vi "Lab Panel V5.10.vi"() -> ()   [LabVIEW 2013] (continued)
                n1780 = property on="O/I  LAB05-2" class="Bool (strict)"("DisabledEnum"=w3328) -> ()  [unwired: 2 in, 2 out]
                n1781 = property on="O/I  LAB05-1" class="Bool (strict)"("DisabledEnum"=w3329) -> ()  [unwired: 2 in, 2 out]
                n1782 = property on="O/I  LAB04-1" class="Bool (strict)"("DisabledEnum"=w3331) -> ()  [unwired: 2 in, 2 out]
                n1783 = property on="O/I  LAB04-2" class="Bool (strict)"("DisabledEnum"=w3330) -> ()  [unwired: 2 in, 2 out]
                n1784 = property on="O/I  LAB03-2" class="Bool (strict)"("DisabledEnum"=w3332) -> ()  [unwired: 2 in, 2 out]
                n1785 = Not(x=w3337) -> (.not. x?=w3338:bool)
                n1786 = Not(x=w3336) -> (.not. x?=w3339:bool)
                n1787 = Not(x=w3335) -> (.not. x?=w3340:bool)
                n1788 = property on="RESULT LAB05-2" class="Bool (strict)"("Visible"=w3338) -> ()  [unwired: 2 in, 2 out]
                n1789 = property on="RESULT LAB05-1" class="Bool (strict)"("Visible"=w3339) -> ()  [unwired: 2 in, 2 out]
                n1790 = Not(x=w3334) -> (.not. x?=w3341:bool)
                n1791 = property on="RESULT LAB04-2" class="Bool (strict)"("Visible"=w3340) -> ()  [unwired: 2 in, 2 out]
                n1792 = Not(x=w3333) -> (.not. x?=w3342:bool)
                n1793 = property on="RESULT LAB04-1" class="Bool (strict)"("Visible"=w3341) -> ()  [unwired: 2 in, 2 out]
                n1794 = property on="RESULT LAB03-2" class="Bool (strict)"("Visible"=w3342) -> ()  [unwired: 2 in, 2 out]
              }
              frame #2 {
                # "disable calibrate if any test running"
                n1795 = Or(x=w3365, y=w3364) -> (x .or. y?=w3358:bool)
                n1796 = Or(x=w3367, y=w3366) -> (x .or. y?=w3360:bool)
                n1797 = Or(x=w3371, y=w3370) -> (x .or. y?=w3362:bool)
                n1798 = Or(x=w3369, y=w3368) -> (x .or. y?=w3361:bool)
                n1799 = Or(x=w3373, y=w3372) -> (x .or. y?=w3363:bool)
                n1800 = Or(x=w3361, y=w3360) -> (x .or. y?=w3359:bool)
                n1801 = Or(x=w3363, y=w3362) -> (x .or. y?=w3357:bool)
                n1802 = Or(x=w3359, y=w3358) -> (x .or. y?=w3356:bool)
                n1803 = Or(x=w3357, y=w3356) -> (x .or. y?=w3355:bool)
                n1804 = case shown="False" w3355 {
                  tunnel: [0 2] -> w3354
                  frame False {
                  }
                  frame True {
                  }
                }
                n1805 = property on="JIG TEST" class="Clust (strict)"("DisabledEnum"=w3354) -> ()  [unwired: 2 in, 2 out]
                n1806 = property on="Network Directory" class="Path"("DisabledEnum"=w3354) -> ()  [unwired: 2 in, 2 out]
                n1807 = property on="MAIL SETTINGS" class="Clust (strict)"("DisabledEnum"=w3354) -> ()  [unwired: 2 in, 2 out]
                n1808 = property on="SET (cal)" class="Bool (strict)"("DisabledEnum"=w3354) -> ()  [unwired: 2 in, 2 out]
                n1809 = property on="ADMIN" class="Bool (strict)"("DisabledEnum"=0) -> ()  [unwired: 2 in, 2 out]
              }
            }
          }
          frame #8 {
            # "drive jigs"
            n1810 = stacked-sequence {
              frame #0 {
                # "jig on"
                n1811 = local read "jig cycle"() -> (w3381:dbl)
                n1812 = property on="JIG TEST" class="Clust (strict)"() -> ("DisabledEnum"=w3378:T16)  [unwired: 2 in, 2 out]
                n1813 = Equal?(x=w3378, y=2) -> (x = y?=w3377:bool)
                n1814 = Equal?(x=w3381, y=0) -> (x = y?=w3379:bool)
                n1815 = And(x=w3379, y=w3377) -> (x .and. y?=w3376:bool)
                n1816 = case shown="True" w3376 {
                  frame False {
                  }
                  frame True {
                    n1817 = local read "run lab01-1"() -> (w3392:bool)
                    n1818 = local read "run lab01-2"() -> (w3391:bool)
                    n1819 = local read "run lab02-1"() -> (w3390:bool)
                    n1820 = local read "run lab02-2"() -> (w3389:bool)
                    n1821 = local read "run lab03-1"() -> (w3388:bool)
                    n1822 = local read "run lab03-2"() -> (w3387:bool)
                    n1823 = local read "run lab04-1"() -> (w3386:bool)
                    n1824 = local read "run lab04-2"() -> (w3385:bool)
                    n1825 = local read "run lab05-1"() -> (w3384:bool)
                    n1826 = local read "run lab05-2"() -> (w3383:bool)
                    n1827 = local write "JIG LAB03-2"(w3387) -> ()
                    n1828 = local write "JIG LAB01-1"(w3392) -> ()
                    n1829 = local write "JIG LAB01-2"(w3391) -> ()
                    n1830 = local write "JIG LAB02-1"(w3390) -> ()
                    n1831 = local write "JIG LAB02-2"(w3389) -> ()
                    n1832 = local write "JIG LAB03-1"(w3388) -> ()
                    n1833 = local write "JIG LAB04-1"(w3386) -> ()
                    n1834 = local write "JIG LAB04-2"(w3385) -> ()
                    n1835 = local write "JIG LAB05-1"(w3384) -> ()
                    n1836 = local write "JIG LAB05-2"(w3383) -> ()
                  }
                }
              }
              frame #1 {
                # "jig off"
                n1837 = local read "jig cycle"() -> (w3399:dbl)
                n1838 = local read "on loops"() -> (w3398:dbl)
                n1839 = property on="JIG TEST" class="Clust (strict)"() -> ("DisabledEnum"=w3397:T16)  [unwired: 2 in, 2 out]
                n1840 = Equal?(x=w3397, y=2) -> (x = y?=w3395:bool)
                n1841 = Equal?(x=w3399, y=w3398) -> (x = y?=w3394:bool)
                n1842 = And(x=w3394, y=w3395) -> (x .and. y?=w3393:bool)
                n1843 = case shown="True" w3393 {
                  frame False {
                  }
                  frame True {
                    w3450 = FALSE
                    w3451 = TRUE
                    w3449 = 2
                    n1844 = local read "SELECT LAB05-2"() -> (w3440:T3)
                    n1845 = local read "SELECT LAB04-2"() -> (w3442:T3)
                    n1846 = local read "SELECT LAB04-1"() -> (w3443:T3)
                    n1847 = local read "SELECT LAB05-1"() -> (w3441:T3)
                    n1848 = local read "SELECT LAB03-2"() -> (w3444:T3)
                    n1849 = local read "SELECT LAB02-1"() -> (w3447:T3)
                    n1850 = local read "SELECT LAB03-1"() -> (w3445:T3)
                    n1851 = local read "SELECT LAB02-2"() -> (w3446:T3)
                    n1852 = local read "SELECT LAB01-2"() -> (w3448:T3)
                    n1853 = local read "run lab05-1"() -> (w3410:bool)
                    n1854 = local read "run lab05-2"() -> (w3409:bool)
                    n1855 = local read "SELECT LAB01-1"() -> (w3452:T3)
                    n1856 = local read "run lab04-2"() -> (w3411:bool)
                    n1857 = local read "run lab04-1"() -> (w3412:bool)
                    n1858 = local read "run lab01-1"() -> (w3428:bool)
                    n1859 = local read "run lab01-2"() -> (w3417:bool)
                    n1860 = local read "run lab03-2"() -> (w3413:bool)
                    n1861 = local read "run lab03-1"() -> (w3414:bool)
                    n1862 = local read "run lab02-1"() -> (w3416:bool)
                    n1863 = local read "run lab02-2"() -> (w3415:bool)
                    n1864 = Equal?(x=w3449, y=w3445) -> (x = y?=w3423:bool)
                    n1865 = Equal?(x=w3449, y=w3444) -> (x = y?=w3422:bool)
                    n1866 = Equal?(x=w3449, y=w3443) -> (x = y?=w3421:bool)
                    n1867 = Equal?(x=w3449, y=w3442) -> (x = y?=w3420:bool)
                    n1868 = Equal?(x=w3449, y=w3441) -> (x = y?=w3419:bool)
                    n1869 = Equal?(x=w3449, y=w3440) -> (x = y?=w3418:bool)
                    n1870 = Equal?(x=w3449, y=w3452) -> (x = y?=w3429:bool)
                    n1871 = Equal?(x=w3449, y=w3447) -> (x = y?=w3425:bool)
                    n1872 = Equal?(x=w3449, y=w3446) -> (x = y?=w3424:bool)
                    n1873 = Equal?(x=w3449, y=w3448) -> (x = y?=w3426:bool)
                    n1874 = And(x=w3420, y=w3411) -> (x .and. y?=w3402:bool)
                    n1875 = And(x=w3423, y=w3414) -> (x .and. y?=w3405:bool)
                    n1876 = And(x=w3421, y=w3412) -> (x .and. y?=w3403:bool)
                    n1877 = And(x=w3418, y=w3409) -> (x .and. y?=w3400:bool)
                    n1878 = And(x=w3424, y=w3415) -> (x .and. y?=w3406:bool)
                    n1879 = And(x=w3422, y=w3413) -> (x .and. y?=w3404:bool)
                    n1880 = And(x=w3419, y=w3410) -> (x .and. y?=w3401:bool)
                    n1881 = And(x=w3426, y=w3417) -> (x .and. y?=w3408:bool)
                    n1882 = And(x=w3429, y=w3428) -> (x .and. y?=w3427:bool)
                    n1883 = And(x=w3425, y=w3416) -> (x .and. y?=w3407:bool)
                    n1884 = Select(t=w3451, s=w3427, f=w3450) -> (s? t:f=w3430:bool)
                    n1885 = Select(t=w3451, s=w3408, f=w3450) -> (s? t:f=w3431:bool)
                    n1886 = Select(t=w3451, s=w3407, f=w3450) -> (s? t:f=w3432:bool)
                    n1887 = Select(t=w3451, s=w3406, f=w3450) -> (s? t:f=w3433:bool)
                    n1888 = Select(t=w3451, s=w3405, f=w3450) -> (s? t:f=w3434:bool)
                    n1889 = Select(t=w3451, s=w3404, f=w3450) -> (s? t:f=w3435:bool)
                    n1890 = Select(t=w3451, s=w3403, f=w3450) -> (s? t:f=w3436:bool)
                    n1891 = Select(t=w3451, s=w3402, f=w3450) -> (s? t:f=w3437:bool)
                    n1892 = Select(t=w3451, s=w3401, f=w3450) -> (s? t:f=w3438:bool)
                    n1893 = Select(t=w3451, s=w3400, f=w3450) -> (s? t:f=w3439:bool)
                    n1894 = local write "JIG LAB03-2"(w3435) -> ()
                    n1895 = local write "JIG LAB02-1"(w3432) -> ()
                    n1896 = local write "JIG LAB02-2"(w3433) -> ()
                    n1897 = local write "JIG LAB01-2"(w3431) -> ()
                    n1898 = local write "JIG LAB03-1"(w3434) -> ()
                    n1899 = local write "JIG LAB01-1"(w3430) -> ()
                    n1900 = local write "JIG LAB05-2"(w3439) -> ()
                    n1901 = local write "JIG LAB04-1"(w3436) -> ()
                    n1902 = local write "JIG LAB05-1"(w3438) -> ()
                    n1903 = local write "JIG LAB04-2"(w3437) -> ()
                  }
                }
              }
            }
          }
          frame #9 {
            # "enable  jig test output if no test busy"
            n1904 = property on="JIG TEST" class="Clust (strict)"() -> ("DisabledEnum"=w3455:T16)  [unwired: 2 in, 2 out]
            n1905 = Equal?(x=w3455, y=0) -> (x = y?=w3453:bool)
            n1906 = case shown="True" w3453 {
              frame False {
              }
              frame True {
                n1907 = local read "JIG TEST"() -> (w3466:T10)
                n1908 = Unbundle(w3466) -> ("LAB01-1"=w3465:bool, "LAB01-2"=w3464:bool, "LAB02-1"=w3463:bool, "LAB02-2"=w3462:bool, "LAB03-1"=w3461:bool, "LAB03-2"=w3460:bool, "LAB04-1"=w3459:bool, "LAB04-2"=w3458:bool, "LAB05-1"=w3457:bool, "LAB05-2"=w3456:bool)
                n1909 = local write "JIG LAB05-1"(w3457) -> ()
                n1910 = local write "JIG LAB05-2"(w3456) -> ()
                n1911 = local write "JIG LAB04-1"(w3459) -> ()
                n1912 = local write "JIG LAB04-2"(w3458) -> ()
                n1913 = local write "JIG LAB03-2"(w3460) -> ()
                n1914 = local write "JIG LAB01-1"(w3465) -> ()
                n1915 = local write "JIG LAB02-1"(w3463) -> ()
                n1916 = local write "JIG LAB03-1"(w3461) -> ()
                n1917 = local write "JIG LAB01-2"(w3464) -> ()
                n1918 = local write "JIG LAB02-2"(w3462) -> ()
              }
            }
          }
          frame #10 {
            # "Drive digital output and reset USB and temperature network if required."
            n1919 = global read "Global display 3.vi" "cycle O/F"() -> (w3477:bool)
            n1920 = local read "O/I  LAB05-2"() -> (w3470:bool)
            n1921 = local read "O/I  LAB05-1"() -> (w3472:bool)
            n1922 = local read "JIG LAB05-2"() -> (w3469:bool)
            n1923 = local read "O/I  LAB04-2"() -> (w3474:bool)
            n1924 = local read "JIG LAB05-1"() -> (w3471:bool)
            n1925 = local read "JIG LAB04-2"() -> (w3473:bool)
            n1926 = local read "O/I  LAB03-1"() -> (w3488:bool)
            n1927 = local read "O/I  LAB04-1"() -> (w3484:bool)
            n1928 = local read "O/I  LAB02-1"() -> (w3492:bool)
            n1929 = local read "O/I  LAB02-2"() -> (w3490:bool)
            n1930 = local read "O/I  LAB03-2"() -> (w3486:bool)
            n1931 = local read "JIG LAB04-1"() -> (w3483:bool)
            n1932 = local read "JIG LAB03-2"() -> (w3485:bool)
            n1933 = local read "O/I  LAB01-2"() -> (w3494:bool)
            n1934 = local read "JIG LAB02-1"() -> (w3491:bool)
            n1935 = local read "JIG LAB02-2"() -> (w3489:bool)
            n1936 = local read "JIG LAB03-1"() -> (w3487:bool)
            n1937 = local read "O/I  LAB01-1"() -> (w3496:bool)
            n1938 = local read "JIG LAB01-2"() -> (w3493:bool)
            n1939 = local read "JIG LAB01-1"() -> (w3495:bool)
            n1940 = case shown="False" w3477 {
              tunnel: [w3542 FALSE] -> w3476
              frame False {
                n1941 = local read "Analog error"() -> (w3541:bool)
                n1942 = local read "Reset Measuring"() -> (w3540:bool)
                n1943 = Or(x=w3540, y=w3541) -> (x .or. y?=w3542:bool)
              }
              frame True {
              }
            }
            n1944 = Build Array(w3489, w3488, w3487, w3486, w3485, w3484, w3483) -> (w3481:bool[])
            n1945 = Build Array(w3496, w3495, w3494, w3493, w3492, w3491, w3490) -> (w3482:bool[])
            n1946 = Build Array(w3474, w3473, w3472, w3471, w3470, w3469, w3476) -> (w3480:bool[])
            n1947 = Build Array(w3474, w3473, w3472, w3471, w3470, w3469, FALSE) -> (w3467:bool[])
            n1948 = Not(x=w3477) -> (.not. x?=w3478:bool)
            n1949 = local read "simulate"() -> (w3479:bool)
            n1950 = And(x=w3478, y=w3476) -> (x .and. y?=w3475:bool)
            n1951 = stacked-sequence {
              tunnel: w3482 -> [w3500 w3506]
              tunnel: w3481 -> [w3499 w3505]
              tunnel: w3480 -> [w3498 _]
              tunnel: w3479 -> [w3497 w3507]
              tunnel: w3475 -> [_ w3508]
              tunnel: w3467 -> [_ w3504]
              frame #0 {
                n1952 = case shown="False" w3497 {
                  tunnel: w3500 -> [w3503 _]
                  tunnel: w3499 -> [w3502 _]
                  tunnel: w3498 -> [w3501 _]
                  frame False {
                    n1953 = call "sub vi - Drive Relays All v6.vi"("Array #2"=w3501, "Array #1"=w3502, "Array #0"=w3503) -> ()  [unwired: 8 in, 1 out]
                  }
                  frame True {
                  }
                }
              }
              frame #1 {
                n1954 = case shown="True" w3508 {
                  tunnel: w3507 -> [_ w3513]
                  tunnel: w3506 -> [_ w3511]
                  tunnel: w3505 -> [_ w3510]
                  tunnel: w3504 -> [_ w3509]
                  frame False {
                  }
                  frame True {
                    n1955 = stacked-sequence {
                      tunnel: w3513 -> [w3520 _]
                      tunnel: bool[] [] -> [_ w3525]
                      tunnel: w3511 -> [_ w3524]
                      tunnel: w3510 -> [_ w3522]
                      tunnel: w3509 -> [_ w3521]
                      frame #0 {
                        w3516 = FALSE
                        # "reset all usb modules"
                        n1956 = local read "Resets Done"() -> (w3515:dbl)
                        n1957 = call "Reset Meas v 3.vi"("simulate"=w3520) -> ("Error USB #2"=w3517:bool, "Error USB #1"=w3518:bool, "Error USB #0"=w3519:bool)  [unwired: 8 in]
                        n1958 = Increment(x=w3515) -> (x+1=→"Resets Done":dbl)
                        n1959 = local write "Error USB #2"(w3517) -> ()
                        n1960 = local write "Error USB #0"(w3519) -> ()
                        n1961 = local write "Error USB #1"(w3518) -> ()
                        n1962 = local write "Reset Measuring"(w3516) -> ()
                        n1963 = local write "Analog error"(w3516) -> ()
                      }
                      frame #1 {
                        # "switch test stations back on after reset"
                        n1964 = stacked-sequence {
                          tunnel: w3525 -> [w3529 w3532 _]
                          tunnel: w3524 -> [w3528 w3534 w3539]
                          tunnel: 3000 -> [w3527 w3530 w3535]
                          tunnel: w3522 -> [_ w3533 w3538]
                          tunnel: w3521 -> [_ _ w3537]
                          frame #0 {
                            # "drive 1st 7 inputs"
                            n1965 = call "sub vi - Drive Relays All v6.vi"("Array #2"=w3529, "Array #1"=w3529, "Array #0"=w3528) -> ()  [unwired: 8 in, 1 out]
                            n1966 = call "Message Display V1.vi"("Message"="Delay on LAB 01-1 to 02-1", "Delay mS"=w3527) -> ()  [unwired: 10 in]
                          }
                          frame #1 {
                            # "drive 1st & 2nd outputs"
                            n1967 = call "sub vi - Drive Relays All v6.vi"("Array #2"=w3532, "Array #1"=w3533, "Array #0"=w3534) -> ()  [unwired: 8 in, 1 out]
                            n1968 = call "Message Display V1.vi"("Message"="Delay on LAB 02-2 to 04-1", "Delay mS"=w3530) -> ()  [unwired: 10 in]
                          }
                          frame #2 {
                            n1969 = call "sub vi - Drive Relays All v6.vi"("Array #2"=w3537, "Array #1"=w3538, "Array #0"=w3539) -> ()  [unwired: 8 in, 1 out]
                            n1970 = call "Message Display V1.vi"("Message"="Delay on LAB 04-2 to 05-2", "Delay mS"=w3535) -> ()  [unwired: 10 in]
                          }
                        }
                      }
                    }
                  }
                }
              }
            }
          }
          frame #11 {
            # "get all analog values from USB devices"
            n1971 = local read "on loops"() -> (w3550:dbl)
            n1972 = local read "jig cycle"() -> (w3547:dbl)
            n1973 = Add(x=w3550, y=1) -> (x+y=w3548:dbl)
            n1974 = Equal?(x=w3547, y=1) -> (x = y?=w3544:bool)
            n1975 = Equal?(x=w3547, y=w3548) -> (x = y?=w3546:bool)
            n1976 = Or(x=w3544, y=w3546) -> (x .or. y?=w3545:bool)
            n1977 = global write "Global display 3.vi" "cycle O/F"(w3544) -> ()
            n1978 = case shown="True" w3545 {
              tunnel: w3544 -> [_ w3554]
              frame False {
              }
              frame True {
                n1979 = local read "simulate"() -> (w3557:bool)
                n1980 = case shown="False" w3557 {
                  tunnel: [w3573 0.3 ("Analog loop time")] -> w3564
                  tunnel: [w3572 dynamicdata[] [] ("array GRAPH")] -> w3563
                  tunnel: [w3571 w3578] -> w3562
                  tunnel: [w3570 w3578] -> w3561
                  tunnel: [w3569 w3578] -> w3560
                  tunnel: [w3568 w3578] -> w3559
                  tunnel: [w3567 w3578] -> w3558
                  tunnel: w3554 -> [_ w3582]
                  tunnel: [w3566 "Ambient Volts"] -> w3553
                  tunnel: [w3565 bool[] []] -> w3552
                  frame False {
                    n1981 = call "sub vi - Read Analog All v9.2.vi"() -> ("Analog loop time"=w3573:dbl, "array GRAPH"=w3572:dynamicdata[], "LAB01"=w3571:T26, "LAB02"=w3570:T27, "LAB03"=w3569:T28, "LAB04"=w3568:T29, "deg C"=w3566:dbl, "USB Error"=w3565:bool[], "LAB05"=w3567:T30)  [unwired: 7 in]
                  }
                  frame True {
                    n1982 = local read "ON amps"() -> (w3576:dbl)
                    n1983 = local read "OFF amps"() -> (w3577:dbl)
                    n1984 = local read "VOLTS"() -> (w3580:dbl)
                    n1985 = local read "PF"() -> (w3579:dbl)
                    n1986 = Select(t=w3576, s=w3582, f=w3577) -> (s? t:f=w3581:dbl)
                    n1987 = Bundle("OFF amps"=w3581, "VOLTS"=w3580, "PF"=w3579, "OFF amps"=w3581, "VOLTS"=w3580, "PF"=w3579) -> (w3578:T31)  [unwired: 1 in]
                  }
                }
                n1988 = local read "simulate"() -> (w3556:bool)
                n1989 = stacked-sequence {
                  tunnel: w3564 -> [w3597 _ _ _ _ _ _]
                  tunnel: w3563 -> [w3594 _ _ _ _ _ _]
                  tunnel: w3562 -> [_ w3644 _ _ _ _ _]
                  tunnel: w3561 -> [_ _ w3651 _ _ _ _]
                  tunnel: w3560 -> [_ _ _ w3680 _ _ _]
                  tunnel: w3559 -> [_ _ _ _ w3707 _ _]
                  tunnel: w3558 -> [_ _ _ _ _ w3736 _]
                  tunnel: w3556 -> [_ w3622 w3650 w3678 w3706 w3734 w3765]
                  tunnel: T14 {"1  (A) cal"=1.0, "1 (V) cal"=1.0, "1 (PF) cal"=1.0, "1 (TL) cal"=1.0, "1 (TN) cal"=1.0, "2 (A) cal"=1.0, "2 (V) cal"=1.0, "2 (PF) cal"=1.0, "2 (TL) cal"=1.0, "2 (TN) cal"=1.0} ("CAL LAB01") -> [_ w3621 w3649 w3677 w3705 w3733 _]
                  tunnel: w3553 -> [_ _ _ _ _ _ w3763]
                  tunnel: w3552 -> [w3593 _ _ _ _ _ _]
                  frame #0 {
                    n1990 = Index Array(array=w3593, index=2) -> (element=w3586:bool)
                    n1991 = Index Array(array=w3593, index=1) -> (element=w3588:bool)
                    n1992 = Index Array(array=w3593, index=0) -> (element=w3589:bool)
                    n1993 = local write "AI"(TRUE) -> ()
                    n1994 = Or(x=w3589, y=w3588) -> (x .or. y?=w3587:bool)
                    n1995 = local write "Error USB #2"(w3586) -> ()
                    n1996 = local write "Error USB #0"(w3589) -> ()
                    n1997 = local write "Error USB #1"(w3588) -> ()
                    n1998 = Or(x=w3587, y=w3586) -> (x .or. y?=→"Analog error":bool)
                    n1999 = global write "Global 1.vi" "RATE(Hz)"("RATE (Hz)") -> ()
                    n2000 = global write "Global 1.vi" "SAMPLES"("SAMPLES") -> ()
                    n2001 = Index Array(array=w3594, index=6) -> (element=→"LAB04-1 (GRAPH)":dynamicdata)
                    n2002 = Index Array(array=w3594, index=7) -> (element=→"LAB04-2 (GRAPH)":dynamicdata)
                    n2003 = Index Array(array=w3594, index=9) -> (element=→"LAB05-2 (GRAPH)":dynamicdata)
                    n2004 = Index Array(array=w3594, index=8) -> (element=→"LAB05-1 (GRAPH)":dynamicdata)
                    n2005 = Index Array(array=w3594, index=5) -> (element=→"LAB03-2 (GRAPH)":dynamicdata)
                    n2006 = Index Array(array=w3594, index=0) -> (element=→"LAB01-1 (GRAPH)":dynamicdata)
                    n2007 = Index Array(array=w3594, index=1) -> (element=→"LAB01-2 (GRAPH)":dynamicdata)
                    n2008 = Index Array(array=w3594, index=2) -> (element=→"LAB02-1 (GRAPH)":dynamicdata)
                    n2009 = Index Array(array=w3594, index=3) -> (element=→"LAB02-2 (GRAPH)":dynamicdata)
                    n2010 = Index Array(array=w3594, index=4) -> (element=→"LAB03-1 (GRAPH)":dynamicdata)
                    "AI loop time" <- w3597
                  }
                  frame #1 {
                    n2011 = case shown="False" w3622 {
                      tunnel: [w3645 w3646] -> w3643
                      tunnel: w3621 -> [_ w3646]
                      frame False {
                        n2012 = local read "CAL LAB01"() -> (w3645:T14)
                      }
                      frame True {
                      }
                    }
                    n2013 = Unbundle By Name(w3644) -> ("OFF amps"=w3642:dbl, "VOLTS"=w3641:dbl, "PF"=w3640:dbl, "OFF amps"=w3639:dbl, "VOLTS"=w3638:dbl, "PF"=w3637:dbl)
                    n2014 = Unbundle By Name(w3643) -> ("1  (A) cal"=w3636:dbl, "1 (V) cal"=w3635:dbl, "1 (PF) cal"=w3634:dbl, "2 (A) cal"=w3633:dbl, "2 (V) cal"=w3632:dbl, "2 (PF) cal"=w3631:dbl)  [unwired: 4 out]
                    n2015 = Multiply(x=w3642, y=w3636) -> (x*y=w3629:dbl)
                    n2016 = Multiply(x=w3641, y=w3635) -> (x*y=w3628:dbl)
                    n2017 = Multiply(x=w3640, y=w3634) -> (x*y=w3627:dbl)
                    n2018 = Multiply(x=w3639, y=w3633) -> (x*y=w3625:dbl)
                    n2019 = Multiply(x=w3638, y=w3632) -> (x*y=w3624:dbl)
                    n2020 = Multiply(x=w3637, y=w3631) -> (x*y=w3623:dbl)
                    n2021 = local read "SIG LAB01-1"() -> (w3630:T2)
                    n2022 = local read "SIG LAB01-2"() -> (w3626:T2)
                    n2023 = Bundle By Name(cluster=w3630, "AMPS"=w3629, "VOLTS"=w3628, "PF"=w3627) -> (w3620:T2)
                    n2024 = Bundle By Name(cluster=w3626, "AMPS"=w3625, "VOLTS"=w3624, "PF"=w3623) -> (w3619:T2)
                    n2025 = global write "Global display 1.vi" "SIG LAB01-2"(w3619) -> ()
                    n2026 = global write "Global display 1.vi" "SIG LAB01-1"(w3620) -> ()
                    n2027 = local write "SIG LAB01-2"(w3619) -> ()
                    n2028 = local write "SIG LAB01-1"(w3620) -> ()
                  }
                  frame #2 {
                    n2029 = Unbundle By Name(w3651) -> ("OFF amps"=w3671:dbl, "VOLTS"=w3670:dbl, "PF"=w3669:dbl, "OFF amps"=w3668:dbl, "VOLTS"=w3667:dbl, "PF"=w3666:dbl)
                    n2030 = case shown="True" w3650 {
                      tunnel: [w3673 w3674] -> w3672
                      tunnel: w3649 -> [_ w3674]
                      frame False {
                        n2031 = local read "CAL LAB02"() -> (w3673:T15)
                      }
                      frame True {
                      }
                    }
                    n2032 = Unbundle By Name(w3672) -> ("1  (A) cal"=w3665:dbl, "1 (V) cal"=w3664:dbl, "1 (PF) cal"=w3663:dbl, "2 (A) cal"=w3662:dbl, "2 (V) cal"=w3661:dbl, "2 (PF) cal"=w3660:dbl)  [unwired: 4 out]
                    n2033 = Multiply(x=w3671, y=w3665) -> (x*y=w3658:dbl)
                    n2034 = Multiply(x=w3670, y=w3664) -> (x*y=w3657:dbl)
                    n2035 = Multiply(x=w3669, y=w3663) -> (x*y=w3656:dbl)
                    n2036 = Multiply(x=w3668, y=w3662) -> (x*y=w3654:dbl)
                    n2037 = Multiply(x=w3667, y=w3661) -> (x*y=w3653:dbl)
                    n2038 = Multiply(x=w3666, y=w3660) -> (x*y=w3652:dbl)
                    n2039 = local read "SIG LAB02-1"() -> (w3659:T2)
                    n2040 = local read "SIG LAB02-2"() -> (w3655:T2)
                    n2041 = Bundle By Name(cluster=w3659, "AMPS"=w3658, "VOLTS"=w3657, "PF"=w3656) -> (w3648:T2)
                    n2042 = Bundle By Name(cluster=w3655, "AMPS"=w3654, "VOLTS"=w3653, "PF"=w3652) -> (w3647:T2)
                    n2043 = global write "Global display 1.vi" "SIG LAB02-1"(w3648) -> ()
                    n2044 = local write "SIG LAB02-2"(w3647) -> ()
                    n2045 = global write "Global display 1.vi" "SIG LAB02-2"(w3647) -> ()
                    n2046 = local write "SIG LAB02-1"(w3648) -> ()
                  }
                  frame #3 {
                    n2047 = Unbundle By Name(w3680) -> ("OFF amps"=w3699:dbl, "VOLTS"=w3698:dbl, "PF"=w3697:dbl, "OFF amps"=w3696:dbl, "VOLTS"=w3695:dbl, "PF"=w3694:dbl)
                    n2048 = case shown="True" w3678 {
                      tunnel: [w3701 w3702] -> w3700
                      tunnel: w3677 -> [_ w3702]
                      frame False {
                        n2049 = local read "CAL LAB03"() -> (w3701:T14)
                      }
                      frame True {
                      }
                    }
                    n2050 = Unbundle By Name(w3700) -> ("1  (A) cal"=w3693:dbl, "1 (V) cal"=w3692:dbl, "1 (PF) cal"=w3691:dbl, "2 (A) cal"=w3690:dbl, "2 (V) cal"=w3689:dbl, "2 (PF) cal"=w3688:dbl)  [unwired: 4 out]
                    n2051 = Multiply(x=w3699, y=w3693) -> (x*y=w3686:dbl)
                    n2052 = Multiply(x=w3698, y=w3692) -> (x*y=w3679:dbl)
                    n2053 = Multiply(x=w3697, y=w3691) -> (x*y=w3685:dbl)
                    n2054 = Multiply(x=w3696, y=w3690) -> (x*y=w3683:dbl)
                    n2055 = Multiply(x=w3695, y=w3689) -> (x*y=w3682:dbl)
                    n2056 = Multiply(x=w3694, y=w3688) -> (x*y=w3681:dbl)
                    n2057 = local read "SIG LAB03-1"() -> (w3687:T2)
                    n2058 = local read "SIG LAB03-2"() -> (w3684:T2)
                    n2059 = Bundle By Name(cluster=w3687, "AMPS"=w3686, "VOLTS"=w3679, "PF"=w3685) -> (w3676:T2)
                    n2060 = Bundle By Name(cluster=w3684, "AMPS"=w3683, "VOLTS"=w3682, "PF"=w3681) -> (w3675:T2)
                    n2061 = global write "Global display 1.vi" "SIG LAB03-1"(w3676) -> ()
                    n2062 = global write "Global display 1.vi" "SIG LAB03-2"(w3675) -> ()
                    n2063 = local write "SIG LAB03-2"(w3675) -> ()
                    n2064 = local write "SIG LAB03-1"(w3676) -> ()
                  }
                  frame #4 {
                    n2065 = Unbundle By Name(w3707) -> ("OFF amps"=w3727:dbl, "VOLTS"=w3726:dbl, "PF"=w3725:dbl, "OFF amps"=w3724:dbl, "VOLTS"=w3723:dbl, "PF"=w3722:dbl)
                    n2066 = case shown="False" w3706 {
                      tunnel: [w3729 w3730] -> w3728
                      tunnel: w3705 -> [_ w3730]
                      frame False {
                        n2067 = local read "CAL LAB04"() -> (w3729:T14)
                      }
                      frame True {
                      }
                    }
                    n2068 = Unbundle By Name(w3728) -> ("1  (A) cal"=w3721:dbl, "1 (V) cal"=w3720:dbl, "1 (PF) cal"=w3719:dbl, "2 (A) cal"=w3718:dbl, "2 (V) cal"=w3717:dbl, "2 (PF) cal"=w3716:dbl)  [unwired: 4 out]
                    n2069 = Multiply(x=w3727, y=w3721) -> (x*y=w3714:dbl)
                    n2070 = Multiply(x=w3726, y=w3720) -> (x*y=w3713:dbl)
                    n2071 = Multiply(x=w3725, y=w3719) -> (x*y=w3712:dbl)
                    n2072 = Multiply(x=w3724, y=w3718) -> (x*y=w3710:dbl)
                    n2073 = Multiply(x=w3723, y=w3717) -> (x*y=w3709:dbl)
                    n2074 = Multiply(x=w3722, y=w3716) -> (x*y=w3708:dbl)
                    n2075 = local read "SIG LAB04-1"() -> (w3715:T2)
                    n2076 = local read "SIG LAB04-2"() -> (w3711:T2)
                    n2077 = Bundle By Name(cluster=w3715, "AMPS"=w3714, "VOLTS"=w3713, "PF"=w3712) -> (w3704:T2)
                    n2078 = Bundle By Name(cluster=w3711, "AMPS"=w3710, "VOLTS"=w3709, "PF"=w3708) -> (w3703:T2)
                    n2079 = global write "Global display 1.vi" "SIG LAB04-2"(w3703) -> ()
                    n2080 = global write "Global display 1.vi" "SIG LAB04-1"(w3704) -> ()
                    n2081 = local write "SIG LAB04-2"(w3703) -> ()
                    n2082 = local write "SIG LAB04-1"(w3704) -> ()
                  }
                  frame #5 {
                    n2083 = Unbundle By Name(w3736) -> ("OFF amps"=w3755:dbl, "VOLTS"=w3735:dbl, "PF"=w3754:dbl, "OFF amps"=w3753:dbl, "VOLTS"=w3752:dbl, "PF"=w3751:dbl)
                    n2084 = case shown="False" w3734 {
                      tunnel: [w3757 w3758] -> w3756
                      tunnel: w3733 -> [_ w3758]
                      frame False {
                        n2085 = local read "CAL LAB05"() -> (w3757:T14)
                      }
                      frame True {
                      }
                    }
                    n2086 = Unbundle By Name(w3756) -> ("1  (A) cal"=w3750:dbl, "1 (V) cal"=w3749:dbl, "1 (PF) cal"=w3748:dbl, "2 (A) cal"=w3747:dbl, "2 (V) cal"=w3746:dbl, "2 (PF) cal"=w3745:dbl)  [unwired: 4 out]
                    n2087 = Multiply(x=w3755, y=w3750) -> (x*y=w3743:dbl)
                    n2088 = Multiply(x=w3735, y=w3749) -> (x*y=w3742:dbl)
                    n2089 = Multiply(x=w3754, y=w3748) -> (x*y=w3741:dbl)
                    n2090 = Multiply(x=w3753, y=w3747) -> (x*y=w3739:dbl)
                    n2091 = Multiply(x=w3752, y=w3746) -> (x*y=w3738:dbl)
                    n2092 = Multiply(x=w3751, y=w3745) -> (x*y=w3737:dbl)
                    n2093 = local read "SIG LAB05-1"() -> (w3744:T2)
                    n2094 = local read "SIG LAB05-2"() -> (w3740:T2)
                    n2095 = Bundle By Name(cluster=w3744, "AMPS"=w3743, "VOLTS"=w3742, "PF"=w3741) -> (w3732:T2)
                    n2096 = Bundle By Name(cluster=w3740, "AMPS"=w3739, "VOLTS"=w3738, "PF"=w3737) -> (w3731:T2)
                    n2097 = global write "Global display 1.vi" "SIG LAB05-1"(w3732) -> ()
                    n2098 = global write "Global display 1.vi" "SIG LAB05-2"(w3731) -> ()
                    n2099 = local write "SIG LAB05-2"(w3731) -> ()
                    n2100 = local write "SIG LAB05-1"(w3732) -> ()
                  }
                  frame #6 {
                    # "update ambient referance temperature"
                    n2101 = case shown="True" w3765 {
                      tunnel: [w3768 100.0] -> w3767
                      frame False {
                        n2102 = local read "TEMP REF cal"() -> (w3768:dbl)
                      }
                      frame True {
                      }
                    }
                    n2103 = Less?(x=w3763, y=1) -> (x < y?=w3760:bool)
                    n2104 = Greater?(x=w3763, y=4) -> (0:w3761:bool)
                    n2105 = Or(x=w3760, y=w3761) -> ()  [unwired: 1 out]
                    n2106 = local read "Panel #"() -> (w3766:dbl)
                    n2107 = local write "Analog error"(FALSE) -> ()
                    n2108 = case shown="1" w3766 {
                      tunnel: w3767 -> [_ w3774]
                      tunnel: w3763 -> [_ w3773]
                      frame 0, Default {
                      }
                      frame 1 {
                        n2109 = Multiply(x=w3774, y=w3773) -> (x*y=w3772:dbl)
                        n2110 = Subtract(x=w3772, y=272) -> (x-y=w3770:dbl)
                        "Amb Tp" <- w3770
                        n2111 = local write "Ref deg C"(w3770) -> ()
                      }
                    }
                    "deg C (volts)" <- w3763
                  }
                }
              }
            }
          }
          frame #12 {
            # "save test data to file"
            n2112 = Get Date/Time In Seconds() -> (seconds since 1Jan1904=w3775:timestamp)
            "File Time Stamp" <- w3775
            n2113 = local read "on loops"() -> (w3794:dbl)
            n2114 = local read "jig cycle"() -> (w3791:dbl)
            n2115 = Format Date/Time String(time format string (%c)="%H:%M%:%S", seconds (now)=w3775) -> (date/time string=w3779:string)  [unwired: 1 in]
            n2116 = Add(x=w3794, y=2) -> (x+y=w3792:dbl)
            n2117 = Build Array(w3779) -> (w3778:string[])
            n2118 = Equal?(x=w3791, y=1) -> (x = y?=w3777:bool)
            n2119 = Equal?(x=w3791, y=w3792) -> (x = y?=w3776:bool)
            n2120 = stacked-sequence {
              tunnel: w3790 -> [w3800 _ _ _ _ _ _ _ _ _]
              tunnel: w3789 -> [_ w3876 _ _ _ _ _ _ _ _]
              tunnel: w3788 -> [_ _ w3956 _ _ _ _ _ _ _]
              tunnel: w3787 -> [_ _ _ w4036 _ _ _ _ _ _]
              tunnel: w3786 -> [_ _ _ _ w4116 _ _ _ _ _]
              tunnel: w3785 -> [_ _ _ _ _ w4196 _ _ _ _]
              tunnel: w3784 -> [_ _ _ _ _ _ w4276 _ _ _]
              tunnel: w3783 -> [_ _ _ _ _ _ _ w4356 _ _]
              tunnel: w3782 -> [_ _ _ _ _ _ _ _ w4436 _]
              tunnel: w3781 -> [_ _ _ _ _ _ _ _ _ w4516]
              tunnel: w3778 -> [w3799 w3880 w3960 w4040 w4120 w4200 w4280 w4360 w4440 w4520]
              tunnel: w3777 -> [w3798 w3879 w3959 w4039 w4119 w4199 w4279 w4359 w4439 w4519]
              tunnel: w3776 -> [w3797 w3878 w3958 w4038 w4118 w4198 w4278 w4358 w4438 w4518]
              tunnel: w3775 -> [w3796 w3877 w3957 w4037 w4117 w4197 w4277 w4357 w4437 w4517]
              frame #0 {
                n2121 = case shown="True" w3800 {
                  tunnel: w3799 -> [_ w3805]
                  tunnel: w3798 -> [_ w3804]
                  tunnel: w3797 -> [_ w3802]
                  tunnel: w3796 -> [_ w3801]
                  frame False {
                  }
                  frame True {
                    n2122 = local read "DISP LAB01-1"() -> (w3806:T4)
                    n2123 = local read "SIG LAB01-1"() -> (w3807:T2)
                    n2124 = local read "ON L01-1"() -> (w3803:cluster{"amps":dbl, "volts":dbl, "pf":dbl})
                    n2125 = Unbundle(w3807) -> ("AMPS"=w3813:dbl, "VOLTS"=w3811:dbl, "PF"=w3810:dbl, "Tmp Live"=w3809:dbl, "Tmp Neut"=w3812:dbl)
                    n2126 = Unbundle(w3806) -> ("CYCLE"=w3808:dbl)  [unwired: 2 out]
                    n2127 = stacked-sequence {
                      tunnel: w3813 -> [w3817 w3836]
                      tunnel: w3812 -> [_ w3835]
                      tunnel: w3811 -> [w3816 w3834]
                      tunnel: w3810 -> [w3815 w3833]
                      tunnel: w3809 -> [_ w3832]
                      tunnel: w3808 -> [_ w3831]
                      tunnel: w3805 -> [_ w3830]
                      tunnel: w3804 -> [w3818 _]
                      tunnel: w3803 -> [w3814 w3828]
                      tunnel: w3802 -> [_ w3829]
                      tunnel: w3801 -> [_ w3824]
                      frame #0 {
                        n2128 = case shown="True" w3818 {
                          tunnel: w3817 -> [_ w3823]
                          tunnel: w3816 -> [_ w3822]
                          tunnel: w3815 -> [_ w3821]
                          tunnel: w3814 -> [_ w3819]
                          frame False {
                          }
                          frame True {
                            n2129 = Bundle(cluster=w3819, "amps"=w3823, "volts"=w3822, "pf"=w3821) -> (w3820:cluster{"amps":dbl, "volts":dbl, "pf":dbl})
                            n2130 = local write "ON L01-1"(w3820) -> ()
                          }
                        }
                      }
                      frame #1 {
                        n2131 = Unbundle(w3828) -> ("amps"=w3827:dbl, "volts"=w3826:dbl, "pf"=w3825:dbl)
                        n2132 = case shown="True" w3829 {
                          tunnel: w3836 -> [_ w3837]
                          tunnel: w3835 -> [_ w3875]
                          tunnel: w3834 -> [_ _]
                          tunnel: w3833 -> [_ _]
                          tunnel: w3832 -> [_ w3874]
                          tunnel: w3831 -> [_ w3873]
                          tunnel: w3830 -> [_ w3841]
                          tunnel: w3827 -> [_ w3838]
                          tunnel: w3826 -> [_ w3870]
                          tunnel: w3825 -> [_ w3869]
                          tunnel: w3824 -> [_ w3839]
                          frame False {
                          }
                          frame True {
                            n2133 = local read "TDMS LAB01-1"() -> (w3872:refnum<k34>)
                            n2134 = Build Array(w3870) -> (w3866:dbl[])
                            n2135 = Build Array(w3869) -> (w3865:dbl[])
                            n2136 = Build Array(w3874) -> (w3864:dbl[])
                            n2137 = Build Array(w3875) -> (w3863:dbl[])
                            n2138 = Build Array(w3838) -> (w3868:dbl[])
                            n2139 = Build Array(w3837) -> (w3867:dbl[])
                            n2140 = Build Array(w3873) -> (w3862:dbl[])
                            n2141 = Build Array("AMPS ON", "AMPS OFF", "VOLTS", "PF", "TEMP Live", "TEMP Neut", "CYCLE") -> (w3846:string[])
                            n2142 = Bundle By Name("Y"=w3868, "t0"=w3839) -> (w3861:waveform(dbl))  [unwired: 1 in]
                            n2143 = Bundle By Name("Y"=w3867, "t0"=w3839) -> (w3860:waveform(dbl))  [unwired: 1 in]
                            n2144 = Bundle By Name("Y"=w3866, "t0"=w3839) -> (w3859:waveform(dbl))  [unwired: 1 in]
                            n2145 = Bundle By Name("Y"=w3865, "t0"=w3839) -> (w3858:waveform(dbl))  [unwired: 1 in]
                            n2146 = Bundle By Name("Y"=w3864, "t0"=w3839) -> (w3857:waveform(dbl))  [unwired: 1 in]
                            n2147 = Bundle By Name("Y"=w3863, "t0"=w3839) -> (w3856:waveform(dbl))  [unwired: 1 in]
                            n2148 = Bundle By Name("Y"=w3862, "t0"=w3839) -> (w3855:waveform(dbl))  [unwired: 1 in]
                            n2149 = Build Array(w3861, w3860, w3859, w3858, w3857, w3856, w3855) -> (w3854:waveform(dbl)[])
                            n2150 = TDMS Write(0:w3872, 5:"TEST VALUES", 7:w3846, 9:w3854) -> (4:w3845:refnum<k34>, 6:w3844:string, 15:w3843:errorcluster)  [unwired: 2 in, 1 out]
                            n2151 = TDMS Write(0:w3845, 5:w3844, 7:"TIME", 9:w3841, 11:w3843) -> (15:w3840:errorcluster)  [unwired: 1 in, 3 out]
                            n2152 = local write "data file error"(w3840) -> ()
                          }
                        }
                      }
                    }
                  }
                }
              }
              frame #1 {
                n2153 = case shown="True" w3876 {
                  tunnel: w3880 -> [_ w3885]
                  tunnel: w3879 -> [_ w3884]
                  tunnel: w3878 -> [_ w3882]
                  tunnel: w3877 -> [_ w3881]
                  frame False {
                  }
                  frame True {
                    n2154 = local read "DISP LAB01-2"() -> (w3886:T4)
                    n2155 = local read "SIG LAB01-2"() -> (w3887:T2)
                    n2156 = local read "ON L01-2"() -> (w3883:cluster{"amps":dbl, "volts":dbl, "pf":dbl})
                    n2157 = Unbundle(w3887) -> ("AMPS"=w3893:dbl, "VOLTS"=w3891:dbl, "PF"=w3890:dbl, "Tmp Live"=w3889:dbl, "Tmp Neut"=w3892:dbl)
                    n2158 = Unbundle(w3886) -> ("CYCLE"=w3888:dbl)  [unwired: 2 out]
                    n2159 = stacked-sequence {
                      tunnel: w3893 -> [w3897 w3916]
                      tunnel: w3892 -> [_ w3915]
                      tunnel: w3891 -> [w3896 w3914]
                      tunnel: w3890 -> [w3895 w3913]
                      tunnel: w3889 -> [_ w3912]
                      tunnel: w3888 -> [_ w3911]
                      tunnel: w3885 -> [_ w3910]
                      tunnel: w3884 -> [w3898 _]
                      tunnel: w3883 -> [w3894 w3908]
                      tunnel: w3882 -> [_ w3909]
                      tunnel: w3881 -> [_ w3904]
                      frame #0 {
                        n2160 = case shown="True" w3898 {
                          tunnel: w3897 -> [_ w3903]
                          tunnel: w3896 -> [_ w3902]
                          tunnel: w3895 -> [_ w3901]
                          tunnel: w3894 -> [_ w3899]
                          frame False {
                          }
                          frame True {
                            n2161 = Bundle(cluster=w3899, "amps"=w3903, "volts"=w3902, "pf"=w3901) -> (w3900:cluster{"amps":dbl, "volts":dbl, "pf":dbl})
                            n2162 = local write "ON L01-2"(w3900) -> ()
                          }
                        }
                      }
                      frame #1 {
                        n2163 = Unbundle(w3908) -> ("amps"=w3907:dbl, "volts"=w3906:dbl, "pf"=w3905:dbl)
                        n2164 = case shown="True" w3909 {
                          tunnel: w3916 -> [_ w3948]
                          tunnel: w3915 -> [_ w3955]
                          tunnel: w3914 -> [_ _]
                          tunnel: w3913 -> [_ _]
                          tunnel: w3912 -> [_ w3954]
                          tunnel: w3911 -> [_ w3953]
                          tunnel: w3910 -> [_ w3918]
                          tunnel: w3907 -> [_ w3950]
                          tunnel: w3906 -> [_ w3949]
                          tunnel: w3905 -> [_ w3947]
                          tunnel: w3904 -> [_ w3939]
                          frame False {
                          }
                          frame True {
                            n2165 = local read "TDMS LAB01-2"() -> (w3952:refnum<k34>)
                            n2166 = Build Array(w3949) -> (w3944:dbl[])
                            n2167 = Build Array(w3947) -> (w3943:dbl[])
                            n2168 = Build Array(w3954) -> (w3942:dbl[])
                            n2169 = Build Array(w3955) -> (w3941:dbl[])
                            n2170 = Build Array(w3950) -> (w3946:dbl[])
                            n2171 = Build Array(w3948) -> (w3945:dbl[])
                            n2172 = Build Array(w3953) -> (w3940:dbl[])
                            n2173 = Build Array("AMPS ON", "AMPS OFF", "VOLTS", "PF", "TEMP Live", "TEMP Neut", "CYCLE") -> (w3923:string[])
                            n2174 = Bundle By Name("Y"=w3946, "t0"=w3939) -> (w3938:waveform(dbl))  [unwired: 1 in]
                            n2175 = Bundle By Name("Y"=w3945, "t0"=w3939) -> (w3937:waveform(dbl))  [unwired: 1 in]
                            n2176 = Bundle By Name("Y"=w3944, "t0"=w3939) -> (w3936:waveform(dbl))  [unwired: 1 in]
                            n2177 = Bundle By Name("Y"=w3943, "t0"=w3939) -> (w3935:waveform(dbl))  [unwired: 1 in]
                            n2178 = Bundle By Name("Y"=w3942, "t0"=w3939) -> (w3934:waveform(dbl))  [unwired: 1 in]
                            n2179 = Bundle By Name("Y"=w3941, "t0"=w3939) -> (w3933:waveform(dbl))  [unwired: 1 in]
                            n2180 = Bundle By Name("Y"=w3940, "t0"=w3939) -> (w3932:waveform(dbl))  [unwired: 1 in]
                            n2181 = Build Array(w3938, w3937, w3936, w3935, w3934, w3933, w3932) -> (w3931:waveform(dbl)[])
                            n2182 = TDMS Write(0:w3952, 5:"TEST VALUES", 7:w3923, 9:w3931) -> (4:w3922:refnum<k34>, 6:w3921:string, 15:w3920:errorcluster)  [unwired: 2 in, 1 out]
                            n2183 = TDMS Write(0:w3922, 5:w3921, 7:"TIME", 9:w3918, 11:w3920) -> (15:w3917:errorcluster)  [unwired: 1 in, 3 out]
                            n2184 = local write "data file error"(w3917) -> ()
                          }
                        }
                      }
                    }
                  }
                }
              }
              frame #2 {
                n2185 = case shown="True" w3956 {
                  tunnel: w3960 -> [_ w3965]
                  tunnel: w3959 -> [_ w3964]
                  tunnel: w3958 -> [_ w3962]
                  tunnel: w3957 -> [_ w3961]
                  frame False {
                  }
                  frame True {
                    n2186 = local read "DISP LAB02-1"() -> (w3966:T4)
                    n2187 = local read "SIG LAB02-1"() -> (w3967:T2)
                    n2188 = local read "ON L02-1"() -> (w3963:cluster{"amps":dbl, "volts":dbl, "pf":dbl})
                    n2189 = Unbundle(w3967) -> ("AMPS"=w3973:dbl, "VOLTS"=w3971:dbl, "PF"=w3970:dbl, "Tmp Live"=w3969:dbl, "Tmp Neut"=w3972:dbl)
                    n2190 = Unbundle(w3966) -> ("CYCLE"=w3968:dbl)  [unwired: 2 out]
                    n2191 = stacked-sequence {
                      tunnel: w3973 -> [w3977 w3996]
                      tunnel: w3972 -> [_ w3995]
                      tunnel: w3971 -> [w3976 w3994]
                      tunnel: w3970 -> [w3975 w3993]
                      tunnel: w3969 -> [_ w3992]
                      tunnel: w3968 -> [_ w3991]
                      tunnel: w3965 -> [_ w3990]
                      tunnel: w3964 -> [w3978 _]
                      tunnel: w3963 -> [w3974 w3988]
                      tunnel: w3962 -> [_ w3989]
                      tunnel: w3961 -> [_ w3984]
                      frame #0 {
                        n2192 = case shown="True" w3978 {
                          tunnel: w3977 -> [_ w3983]
                          tunnel: w3976 -> [_ w3982]
                          tunnel: w3975 -> [_ w3981]
                          tunnel: w3974 -> [_ w3979]
                          frame False {
                          }
                          frame True {
                            n2193 = Bundle(cluster=w3979, "amps"=w3983, "volts"=w3982, "pf"=w3981) -> (w3980:cluster{"amps":dbl, "volts":dbl, "pf":dbl})
                            n2194 = local write "ON L02-1"(w3980) -> ()
                          }
                        }
                      }
                      frame #1 {
                        n2195 = Unbundle(w3988) -> ("amps"=w3987:dbl, "volts"=w3986:dbl, "pf"=w3985:dbl)
                        n2196 = case shown="True" w3989 {
                          tunnel: w3996 -> [_ w4028]
                          tunnel: w3995 -> [_ w4035]
                          tunnel: w3994 -> [_ _]
                          tunnel: w3993 -> [_ _]
                          tunnel: w3992 -> [_ w4034]
                          tunnel: w3991 -> [_ w4033]
                          tunnel: w3990 -> [_ w3998]
                          tunnel: w3987 -> [_ w4030]
                          tunnel: w3986 -> [_ w4029]
